vi "dt to velocity.vi"(11 "dt":u32) -> (3 "Velocity (Km/h)":dbl)   [LabVIEW 2016]
doc: "Input\ndt\n\nOutput\nVelocity\n\nTransforms the time between two magnets into a velocity, and uses a median filter to remove some noise."
uses:
  <vilib>/ptbypt/NI_PtbyPt.lvlib
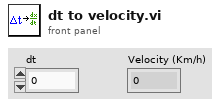
[diagram p1: front panel]
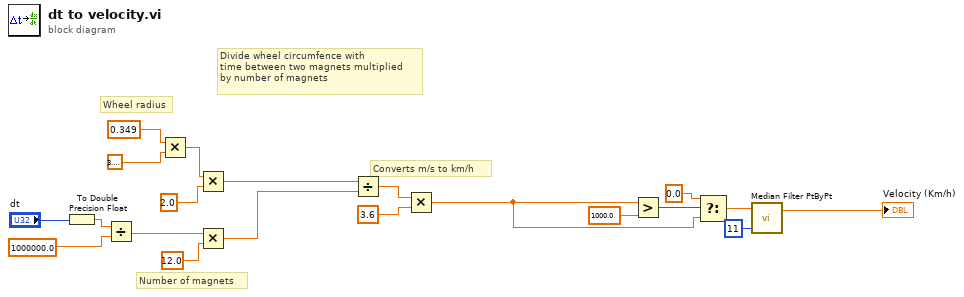
[diagram p0: block diagram]
diagram:
  # "Divide wheel circumfence with\ntime between two magnets multiplied\nby number of magnets"
  # "Wheel radius"
  # "Number of magnets"
  # "Converts m/s to km/h"
  n1 = To Double Precision Float(number="dt") -> (double precision float=w14:dbl)
  n2 = Divide(x=w14, y=1000000.0) -> (x/y=w12:dbl)
  n3 = Multiply(x=0.349, y=3.141592653589793) -> (x*y=w19:dbl)
  n4 = Multiply(x=w19, y=2.0 ("x")) -> (x*y=w16:dbl)
  n5 = Multiply(x=w12, y=12.0) -> (x*y=w15:dbl)
  n6 = Divide(x=w16, y=w15) -> (x/y=w11:dbl)
  n7 = Multiply(x=w11, y=3.6) -> (x*y=w3:dbl)
  n8 = Greater?(x=w3, y=1000.0) -> (0:w4:bool)
  n9 = Select(t=0.0, s=w4, f=w3) -> (s? t:f=w2:dbl)
  n10 = call <vilib>:"Median Filter PtByPt.vi"("rank"=11, "x"=w2) -> ("Filtered x"=→"Velocity (Km/h)":dbl)  [unwired: 2 in, 1 out]
